vi "Top level wrapper ILD1420.vi"(2 "Reconfigure settings":bool, 4 "Data rate (kHz)":string(combo)="0.25", 5 "Auto laser off":bool=TRUE, 6 "Measuring range (mm)":u8(ring)=4 items=["10", "25", "50", "100", "200"], 7 "N samples":i32=2000 min=0) -> (0 "Error out":errorcluster, 1 "d (mm)":dbl[](array[numeric]))   [LabVIEW 2016]
uses:
  Globals/ILD1420_Global.vi
panel:
  # "(set true if changing data rate)"
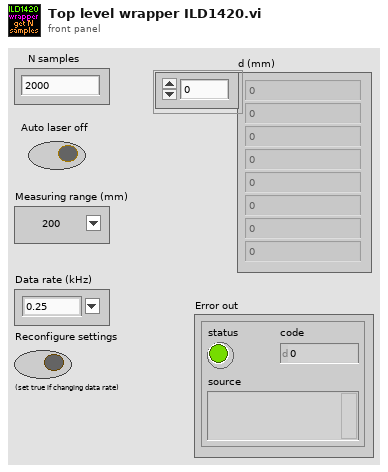
[diagram p1: front panel]
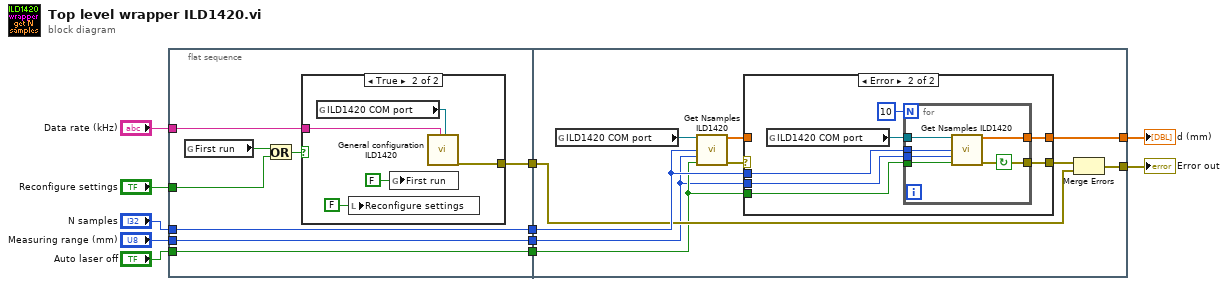
[diagram p0: block diagram]
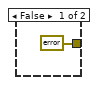
[diagram p2: hidden frame]
diagram:
  n1 = flat-sequence {
    tunnel: "N samples" -> [w19]
    tunnel: [w19] -> w9
    tunnel: [w18] -> w7
    tunnel: [w17] -> w6
    tunnel: "Auto laser off" -> [w17]
    tunnel: [w16] -> w4
    tunnel: "Measuring range (mm)" -> [w16]
    tunnel: "Data rate (kHz)" -> [w15]
    tunnel: "Reconfigure settings" -> [w12]
    tunnel: [w31] -> w11
    tunnel: w9 -> [w32]
    tunnel: [w28] -> w8
    tunnel: w7 -> [w29]
    tunnel: w6 -> [w27]
    tunnel: w4 -> [w26]
    frame #0 {
      n2 = global read "ILD1420_Global.vi" "First run"() -> (w13:bool)
      n3 = Or(x=w13, y=w12) -> (x .or. y?=w14:bool)
      n4 = case shown="True" w14 {
        tunnel: [errorcluster {"status"=FALSE, "code"=0, "source"=""} ("Error out") w23] -> w18
        tunnel: w15 -> [_ w22]
        frame False {
        }
        frame True {
          n5 = global read "ILD1420_Global.vi" "ILD1420 COM port"() -> (w24:refnum<visa-resource-name>)
          n6 = local write "Reconfigure settings"(FALSE ("Reconfigure settings")) -> ()
          n7 = global write "ILD1420_Global.vi" "First run"(FALSE ("First run")) -> ()
          n8 = call "General configuration ILD1420.vi"("Data rate (kHz)"=w22, "COM port"=w24) -> ("Error out"=w23:errorcluster)  [unwired: 17 in]
        }
      }
    }
    frame #1 {
      n9 = global read "ILD1420_Global.vi" "ILD1420 COM port"() -> (w35:refnum<visa-resource-name>)
      n10 = call "Get Nsamples ILD1420.vi"("COM port"=w35, "N samples"=w32, "Measuring range (mm)"=w26, "Auto laser off"=w27) -> ("d (mm)"=w33:dbl[], "Error out"=w34:errorcluster)  [unwired: 10 in]
      n11 = case shown="Error" w34 {
        selector: w34 -> [w36 _]
        tunnel: w33 -> [w37 _]
        tunnel: w32 -> [_ w42]
        tunnel: [w37 w41] -> w31
        tunnel: [w36 w40] -> w30
        tunnel: w27 -> [_ w39]
        tunnel: w26 -> [_ w38]
        frame No Error {
        }
        frame Error {
          n12 = global read "ILD1420_Global.vi" "ILD1420 COM port"() -> (w43:refnum<visa-resource-name>)
          n13 = for {
            N: 10 -> [_]
            tunnel: w43 -> [w50]
            tunnel: w42 -> [w49]
            tunnel: [w48] -> w41
            tunnel: [w47] -> w40
            tunnel: w39 -> [w46]
            tunnel: w38 -> [w45]
            stop <- w47 continue-if-true
            n14 = call "Get Nsamples ILD1420.vi"("COM port"=w50, "N samples"=w49, "Measuring range (mm)"=w45, "Auto laser off"=w46) -> ("d (mm)"=w48:dbl[], "Error out"=w47:errorcluster)  [unwired: 10 in]
          }
        }
      }
      n15 = Merge Errors(w30, w29) -> (w28:errorcluster)
    }
  }
  "d (mm)" <- w11
  "Error out" <- w8
